vi "data create2.vi"(6 "y 3":string="Null", 7 "y":string="Null", 8 "old":string[](array[string]), 9 "y 2":dbl=0.025 format="%#_13g", 10 "索引":i32=1, 11 "new":string[](array[string])) -> (3 "Data":string)   [LabVIEW 2015]
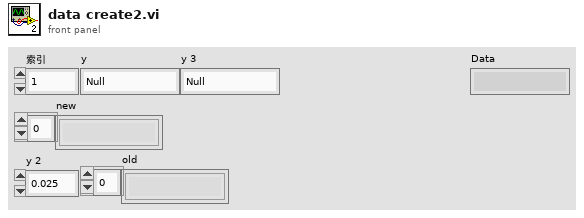
[diagram p1: front panel]
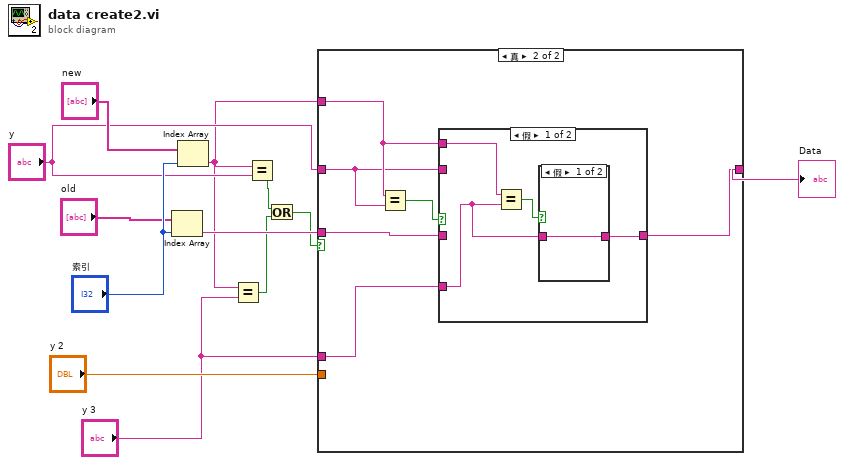
[diagram p0: block diagram]
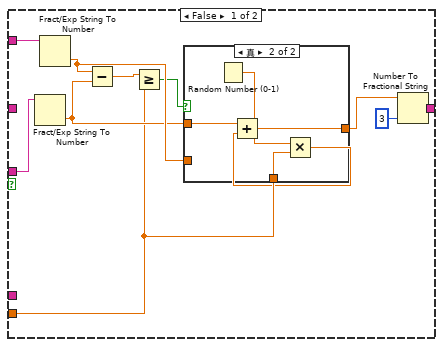
[diagram p2: hidden frame]
diagram:
  n1 = Index Array(array="old", index="索引") -> (element=w11:string)
  n2 = Index Array(array="new", index="索引") -> (element=w5:string)
  n3 = Equal?(x=w5, y="y 3") -> (x = y?=w3:bool)
  n4 = Equal?(x=w5, y="y") -> (x = y?=w4:bool)
  n5 = Or(x=w4, y=w3) -> (x .or. y?=w2:bool)
  n6 = case shown="真" w2 {
    tunnel: w11 -> [w18 w32]
    tunnel: w5 -> [w15 w30]
    tunnel: "y 2" -> [w14 _]
    tunnel: [w13 w33] -> w8
    tunnel: "y" -> [_ w29]
    tunnel: "y 3" -> [_ w31]
    frame False {
      n7 = Fract/Exp String To Number(string=w18) -> (number=w20:dbl)  [unwired: 3 in, 1 out]
      n8 = Fract/Exp String To Number(string=w15) -> (number=w22:dbl)  [unwired: 3 in, 1 out]
      n9 = Subtract(x=w22, y=w20) -> (x-y=w21:dbl)
      n10 = Greater Or Equal?(x=w21, y=w14) -> (x >= y?=w19:bool)
      n11 = case shown="真" w19 {
        tunnel: w20 -> [_ w28]
        tunnel: w22 -> [w23 _]
        tunnel: [w23 w25] -> w16
        tunnel: w14 -> [_ w24]
        frame False {
        }
        frame True {
          n12 = Random Number (0-1)() -> (number: 0 to 1=w27:dbl)
          n13 = Multiply(x=w27, y=w24) -> (x*y=w26:dbl)
          n14 = Add(x=w28, y=w26) -> (x+y=w25:dbl)
        }
      }
      n15 = Number To Fractional String(number=w16, precision (6)=i16 3 ("精度(6)")) -> (F-format string=w13:string)  [unwired: 2 in]
    }
    frame True {
      n16 = Equal?(x=w30, y=w29) -> (x = y?=w34:bool)
      n17 = case shown="假" w34 {
        tunnel: w29 -> [_ w41]
        tunnel: [w35 w41] -> w33
        tunnel: w32 -> [_ _]
        tunnel: w31 -> [w36 _]
        tunnel: w30 -> [w38 _]
        frame False {
          n18 = Equal?(x=w38, y=w36) -> (x = y?=w37:bool)
          n19 = case shown="假" w37 {
            tunnel: w36 -> [w39 w40]
            tunnel: [w39 w40] -> w35
            frame False {
            }
            frame True {
            }
          }
        }
        frame True {
        }
      }
    }
  }
  "Data" <- w8
